vi "Custom Processing.vi"(0 "tagged llp packets cluster in":T1, 1 "reset":bool, 5 "end of data":bool[](array[boolean])=[FALSE, TRUE, TRUE, TRUE, TRUE, TRUE, TRUE, TRUE], 9 "input valid":bool[](array[boolean])=[FALSE, FALSE, FALSE, FALSE, FALSE, FALSE, FALSE, FALSE], 12 "ready for output":bool[](array[boolean])=[TRUE, TRUE, TRUE, TRUE, TRUE, TRUE, TRUE, TRUE]) -> (4 "tagged llp packets cluster out":T1, 6 "end of data out":bool[](array[boolean]), 10 "output valid":bool[](array[boolean]), 14 "ready for input":bool[](array[boolean]))   [LabVIEW 2020, in "GettingStarted_Gen_148X_FPGA.lvlib"]
uses:
  GettingStarted_Gen_148X_FPGA.lvlib
  Common/Types/Tagged LLP Packets Cluster.ctl
  <instrlib>/FlexRIO/CSI-2/v2/FPGA/Types/Tagged LLP Packet.ctl
  <instrlib>/FlexRIO/CSI-2/v2/FPGA/Types/FPGA LLP Packet Tag.ctl
  <instrlib>/FlexRIO/CSI-2/v2/FPGA/Types/FPGA LLP Packet Timestamp.ctl
  <instrlib>/FlexRIO/CSI-2/v2/FPGA/Types/Timestamp ID.ctl
  <instrlib>/FlexRIO/CSI-2/v2/FPGA/Types/FPGA LLP Packet Size.ctl
  <instrlib>/FlexRIO/CSI-2/v2/FPGA/Types/LLP Packet.ctl
  <instrlib>/FlexRIO/CSI-2/v2/FPGA/Types/LLP Packet Header.ctl
  <instrlib>/FlexRIO/CSI-2/v2/FPGA/Types/LLP Packet Payload.ctl
  <instrlib>/FlexRIO/CSI-2/v2/FPGA/Types/LLP Packet Footer.ctl
  <instrlib>/_niInstr/Basic Elements/v1/FPGA/niInstr Basic Elements v1 FPGA.lvlib
  <instrlib>/FlexRIO/CSI-2/v2/FPGA/NI CSI-2 API FPGA v2.lvlib
  Common/GettingStarted_Common_148X_FPGA.lvlib
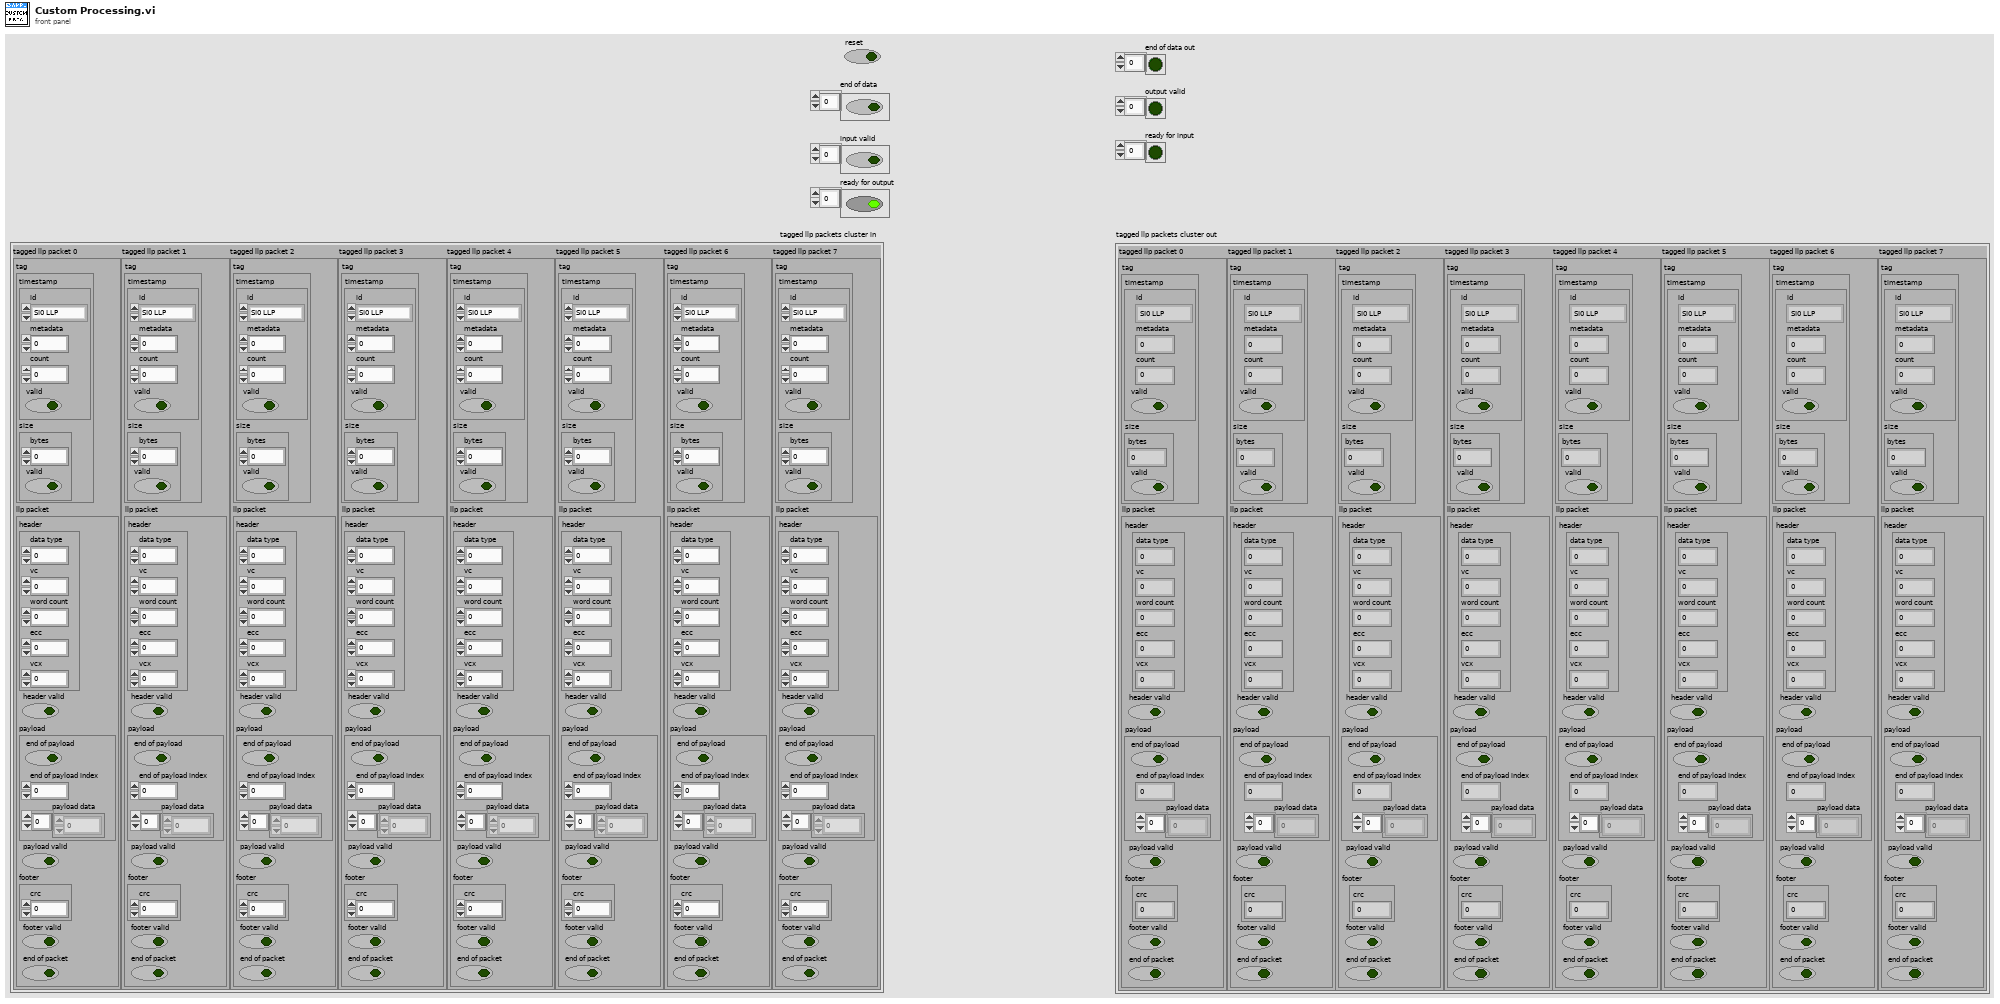
[diagram p1: front panel]
types:
  T1 = typedef "GettingStarted_Common_148X_FPGA.lvlib/Tagged LLP Packets Cluster.ctl" = cluster{"tagged llp packet 0":T2, "tagged llp packet 1":T2, "tagged llp packet 2":T2, "tagged llp packet 3":T2, "tagged llp packet 4":T2, "tagged llp packet 5":T2, "tagged llp packet 6":T2, "tagged llp packet 7":T2}
  T2 = typedef "NI CSI-2 API FPGA v2.lvlib/Tagged LLP Packet.ctl" = cluster{"tag":T3, "llp packet":T7}
  T3 = typedef "NI CSI-2 API FPGA v2.lvlib/FPGA LLP Packet Tag.ctl" = cluster{"timestamp":T4, "size":T6}
  T4 = typedef "NI CSI-2 API FPGA v2.lvlib/FPGA LLP Packet Timestamp.ctl" = cluster{"valid":bool, "count":fxp<+,50,50>, "id":T5, "metadata":u8}
  T5 = typedef "NI CSI-2 API FPGA v2.lvlib/Timestamp ID.ctl" = enum8{"SI0 LLP", "SI1 LLP", "SI2 LLP", "SI3 LLP", "SI4 LLP", "SI5 LLP", "SI6 LLP", "SI7 LLP", "SO0 LLP", "SO1 LLP", "SO2 LLP", "SO3 LLP", "SO4 LLP", "SO5 LLP", "SO6 LLP", "SO7 LLP", "Ser0 GPIO Bank", "Ser1 GPIO Bank", "Ser2 GPIO Bank", "Ser3 GPIO Bank", "Ser4 GPIO Bank", "Ser5 GPIO Bank", "Ser6 GPIO Bank", "Ser7 GPIO Bank", "Des0 GPIO Bank", "Des1 GPIO Bank", "Des2 GPIO Bank", "Des3 GPIO Bank", "Des4 GPIO Bank", "Des5 GPIO Bank", "Des6 GPIO Bank", "Des7 GPIO Bank", "User0", "User1", "User2", "User3", "User4", "User5", "User6", "User7", "User8", "User9", "User10", "User11", "User12", "User13", "User14", "User15", "User16", "User17", "User18", "User19", "User20", "User21", "User22", "User23", "User24", "User25", "User26", "User27", "User28", "User29", "User30", "User31"}
  T6 = typedef "NI CSI-2 API FPGA v2.lvlib/FPGA LLP Packet Size.ctl" = cluster{"bytes":fxp<+,17,17>, "valid":bool}
  T7 = typedef "NI CSI-2 API FPGA v2.lvlib/LLP Packet.ctl" = cluster{"header":T8, "header valid":bool, "payload":T9, "payload valid":bool, "footer":T10, "footer valid":bool, "end of packet":bool}
  T8 = typedef "NI CSI-2 API FPGA v2.lvlib/LLP Packet Header.ctl" = cluster{"word count":u16, "ecc":fxp<+,6,6>, "vcx":fxp<+,2,2>, "data type":fxp<+,6,6>, "vc":fxp<+,2,2>}
  T9 = typedef "NI CSI-2 API FPGA v2.lvlib/LLP Packet Payload.ctl" = cluster{"end of payload":bool, "end of payload index":fxp<+,3,3>, "payload data":u8[]}
  T10 = typedef "NI CSI-2 API FPGA v2.lvlib/LLP Packet Footer.ctl" = cluster{"crc":u16}
  T11 = cluster{"tagged llp packet":T2, "end of data":bool, "input valid":bool, "ready for output":bool}
  T12 = cluster{"end of data out":bool, "output valid":bool, "ready for input":bool}
  T13 = cluster{"end of data out":bool, "output valid":bool, "ready for input":bool}[]
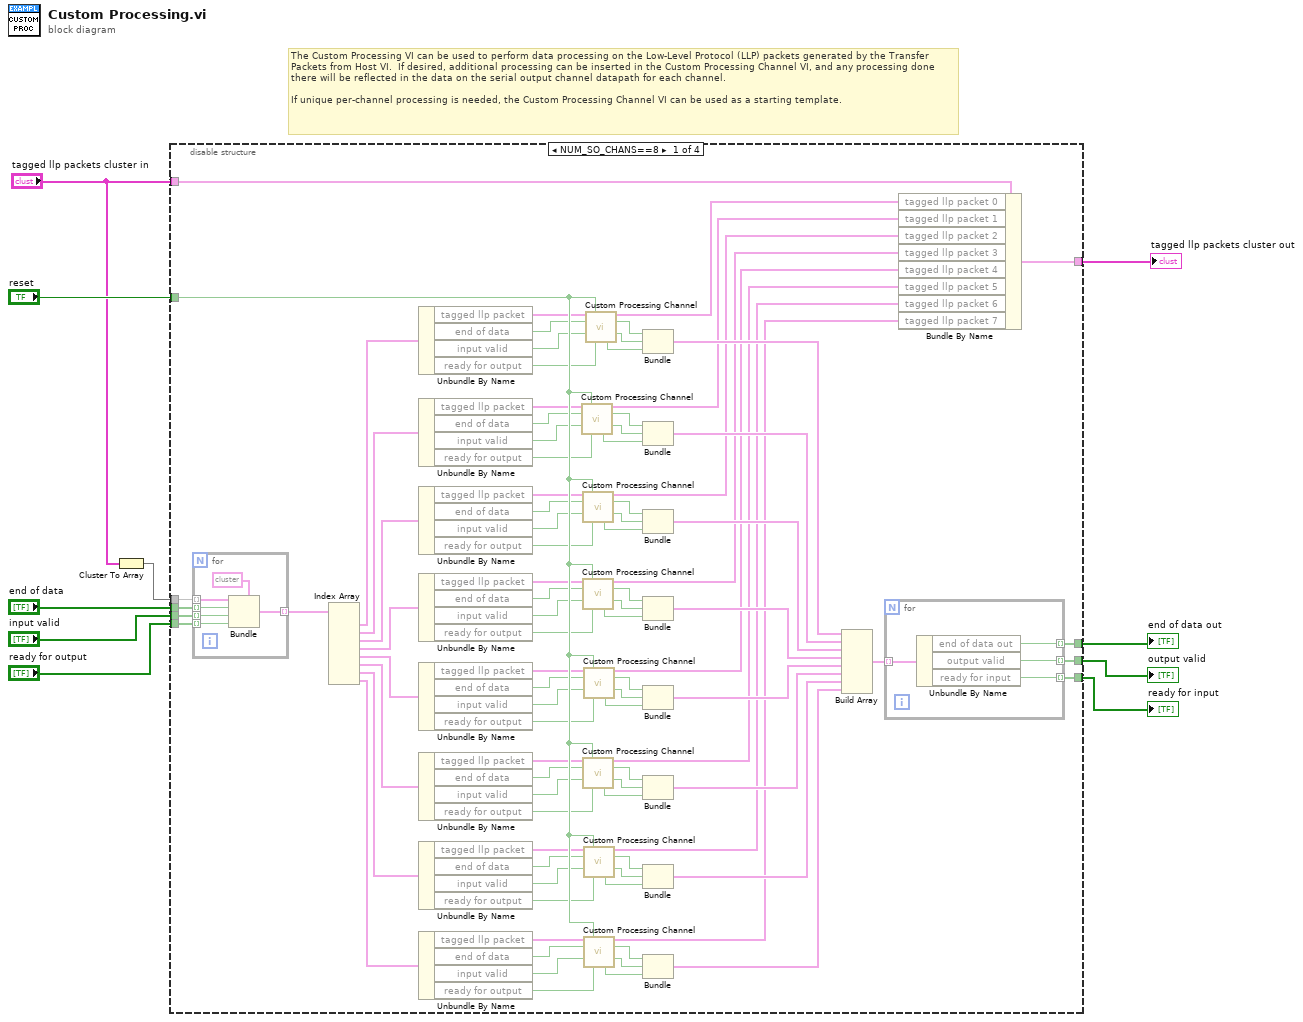
[diagram p0: block diagram]
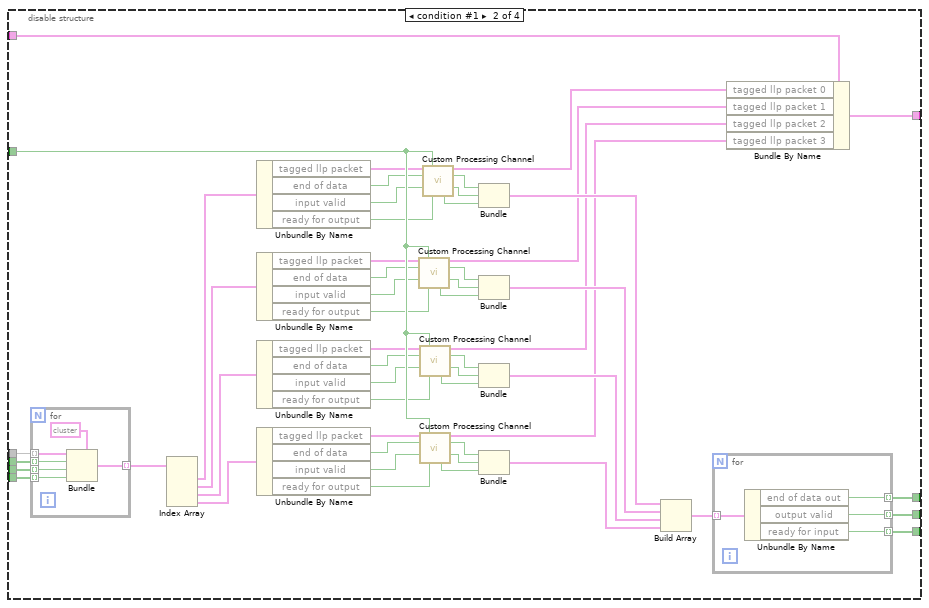
[diagram p2: hidden frame]
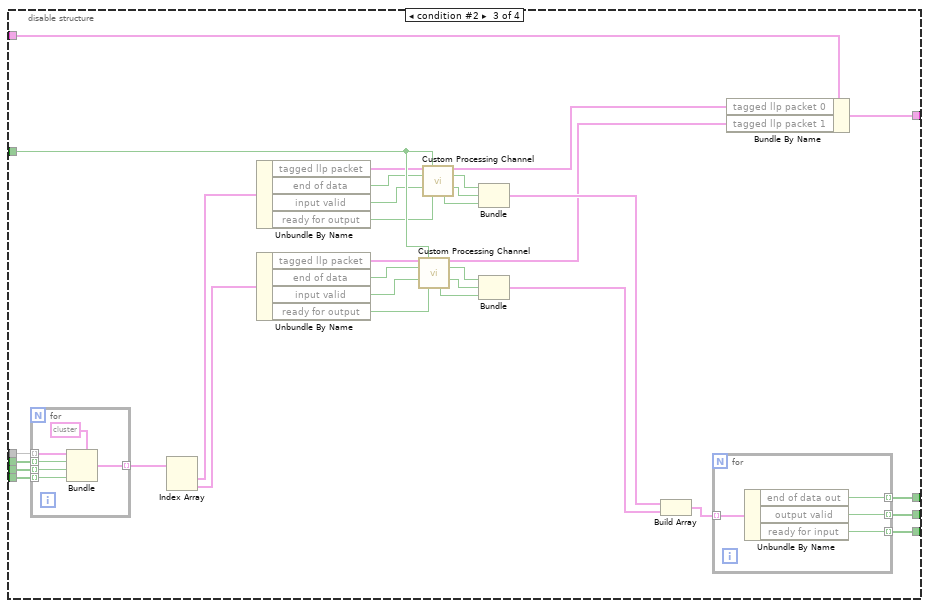
[diagram p3: hidden frame]
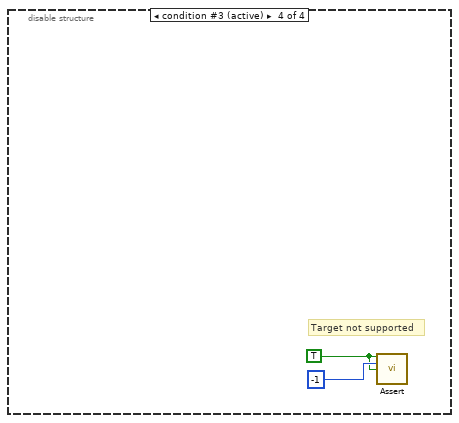
[diagram p4: hidden frame]
diagram:
  # "The Custom Processing VI can be used to perform data processing on the Low-Level Protocol (LLP) packets generated by the Transfer Packets from Host VI.  If desired, additional processing can be inserted in the Custom Processing Channel VI, and any processing done there will be reflected in the data on the serial output channel datapath for each channel.\n\nIf unique per-channel processing is needed, the Custom Processing Channel VI can be used as a starting template."
  n1 = Cluster To Array(cluster="tagged llp packets cluster in") -> (array=w3:T2[])
  n2 = disable-structure shown="NUM_SO_CHANS==8" {
    disable-tunnel: "reset" -> [w91 w158 w202 _]
    disable-tunnel: w3 -> [w102 w114 w176 _]
    disable-tunnel: "end of data" -> [w101 w164 w206 _]
    disable-tunnel: "input valid" -> [w73 w148 w196 _]
    disable-tunnel: "ready for output" -> [w56 w139 w191 _]
    disable-tunnel: [w47 w134 w188 _] -> w4
    disable-tunnel: [w46 w133 w187 _] -> w5
    disable-tunnel: [w21 w120 w180 _] -> w6
    disable-tunnel: [w12 w119 w179 _] -> w2
    disable-tunnel: "tagged llp packets cluster in" -> [w11 w113 w175 _]
    frame condition #0 {
      n3 = for {
        tunnel: w102 -> [w107] mode=indexing
        tunnel: w101 -> [w106] mode=indexing
        tunnel: [w108] -> w100 mode=indexing
        tunnel: w73 -> [w105] mode=indexing
        tunnel: w56 -> [w104] mode=indexing
        n4 = Bundle(cluster=T11 {"tagged llp packet"={"tag"={"timestamp"={"valid"=FALSE, "count"=0.0, "id"=enum."SI0 LLP", "metadata"=0}, "size"={"bytes"=0.0, "valid"=FALSE}}, "llp packet"={"header"={"word count"=0, "ecc"=0.0, "vcx"=0.0, "data type"=0.0, "vc"=0.0}, "header valid"=FALSE, "payload"={"end of payload"=FALSE, "end of payload index"=0.0, "payload data"=[]}, "payload valid"=FALSE, "footer"={"crc"=0}, "footer valid"=FALSE, "end of packet"=FALSE}}, "end of data"=FALSE, "input valid"=FALSE, "ready for output"=FALSE} ("output cluster"), "tagged llp packet"=w107, "end of data"=w106, "input valid"=w105, "ready for output"=w104) -> (w108:T11)
      }
      n5 = Index Array(array=w100) -> (element #1=w99:T11, element #2=w96:T11, element #3=w95:T11, element #4=w93:T11, element #5=w92:T11, element #6=w94:T11, element #7=w97:T11, element #8=w98:T11)  [unwired: 8 in]
      n6 = Unbundle By Name(w99) -> ("tagged llp packet"=w90:T2, "end of data"=w71:bool, "input valid"=w72:bool, "ready for output"=w55:bool)
      n7 = Unbundle By Name(w96) -> ("tagged llp packet"=w89:T2, "end of data"=w70:bool, "input valid"=w69:bool, "ready for output"=w54:bool)
      n8 = Unbundle By Name(w95) -> ("tagged llp packet"=w83:T2, "end of data"=w68:bool, "input valid"=w67:bool, "ready for output"=w53:bool)
      n9 = Unbundle By Name(w93) -> ("tagged llp packet"=w84:T2, "end of data"=w66:bool, "input valid"=w65:bool, "ready for output"=w52:bool)
      n10 = Unbundle By Name(w92) -> ("tagged llp packet"=w85:T2, "end of data"=w64:bool, "input valid"=w63:bool, "ready for output"=w51:bool)
      n11 = Unbundle By Name(w94) -> ("tagged llp packet"=w86:T2, "end of data"=w62:bool, "input valid"=w61:bool, "ready for output"=w50:bool)
      n12 = Unbundle By Name(w97) -> ("tagged llp packet"=w87:T2, "end of data"=w60:bool, "input valid"=w59:bool, "ready for output"=w49:bool)
      n13 = Unbundle By Name(w98) -> ("tagged llp packet"=w88:T2, "end of data"=w58:bool, "input valid"=w57:bool, "ready for output"=w48:bool)
      n14 = call "Custom Processing Channel.vi"("tagged llp packet in"=w89, "reset"=w91, "end of data in"=w70, "input valid"=w69, "ready for output"=w54) -> ("tagged llp packet out"=w14:T2, "end of data out"=w25:bool, "output valid"=w26:bool, "ready for input"=w44:bool)  [unwired: 7 in]
      n15 = call "Custom Processing Channel.vi"("tagged llp packet in"=w83, "reset"=w91, "end of data in"=w68, "input valid"=w67, "ready for output"=w53) -> ("tagged llp packet out"=w15:T2, "end of data out"=w28:bool, "output valid"=w27:bool, "ready for input"=w45:bool)  [unwired: 7 in]
      n16 = call "Custom Processing Channel.vi"("tagged llp packet in"=w84, "reset"=w91, "end of data in"=w66, "input valid"=w65, "ready for output"=w52) -> ("tagged llp packet out"=w16:T2, "end of data out"=w29:bool, "output valid"=w30:bool, "ready for input"=w42:bool)  [unwired: 7 in]
      n17 = call "Custom Processing Channel.vi"("tagged llp packet in"=w86, "reset"=w91, "end of data in"=w62, "input valid"=w61, "ready for output"=w50) -> ("tagged llp packet out"=w18:T2, "end of data out"=w33:bool, "output valid"=w34:bool, "ready for input"=w40:bool)  [unwired: 7 in]
      n18 = call "Custom Processing Channel.vi"("tagged llp packet in"=w85, "reset"=w91, "end of data in"=w64, "input valid"=w63, "ready for output"=w51) -> ("tagged llp packet out"=w17:T2, "end of data out"=w32:bool, "output valid"=w31:bool, "ready for input"=w41:bool)  [unwired: 7 in]
      n19 = call "Custom Processing Channel.vi"("tagged llp packet in"=w87, "reset"=w91, "end of data in"=w60, "input valid"=w59, "ready for output"=w49) -> ("tagged llp packet out"=w19:T2, "end of data out"=w22:bool, "output valid"=w37:bool, "ready for input"=w39:bool)  [unwired: 7 in]
      n20 = call "Custom Processing Channel.vi"("tagged llp packet in"=w88, "reset"=w91, "end of data in"=w58, "input valid"=w57, "ready for output"=w48) -> ("tagged llp packet out"=w20:T2, "end of data out"=w35:bool, "output valid"=w36:bool, "ready for input"=w38:bool)  [unwired: 7 in]
      n21 = call "Custom Processing Channel.vi"("tagged llp packet in"=w90, "reset"=w91, "end of data in"=w71, "input valid"=w72, "ready for output"=w55) -> ("tagged llp packet out"=w13:T2, "end of data out"=w23:bool, "output valid"=w24:bool, "ready for input"=w43:bool)  [unwired: 7 in]
      n22 = Bundle("end of data out"=w23, "output valid"=w24, "ready for input"=w43) -> (w80:T12)  [unwired: 1 in]
      n23 = Bundle("end of data out"=w25, "output valid"=w26, "ready for input"=w44) -> (w77:T12)  [unwired: 1 in]
      n24 = Bundle("end of data out"=w28, "output valid"=w27, "ready for input"=w45) -> (w76:T12)  [unwired: 1 in]
      n25 = Bundle("end of data out"=w29, "output valid"=w30, "ready for input"=w42) -> (w82:T12)  [unwired: 1 in]
      n26 = Bundle("end of data out"=w32, "output valid"=w31, "ready for input"=w41) -> (w81:T12)  [unwired: 1 in]
      n27 = Bundle("end of data out"=w33, "output valid"=w34, "ready for input"=w40) -> (w75:T12)  [unwired: 1 in]
      n28 = Bundle("end of data out"=w22, "output valid"=w37, "ready for input"=w39) -> (w78:T12)  [unwired: 1 in]
      n29 = Bundle("end of data out"=w35, "output valid"=w36, "ready for input"=w38) -> (w79:T12)  [unwired: 1 in]
      n30 = Build Array(w80, w77, w76, w82, w81, w75, w78, w79) -> (w74:T13)
      n31 = for {
        tunnel: w74 -> [w112] mode=indexing
        tunnel: [w111] -> w47 mode=indexing
        tunnel: [w110] -> w46 mode=indexing
        tunnel: [w109] -> w21 mode=indexing
        n32 = Unbundle By Name(w112) -> ("end of data out"=w111:bool, "output valid"=w110:bool, "ready for input"=w109:bool)
      }
      n33 = Bundle By Name(cluster=w11, "tagged llp packet 0"=w13, "tagged llp packet 1"=w14, "tagged llp packet 2"=w15, "tagged llp packet 3"=w16, "tagged llp packet 4"=w17, "tagged llp packet 5"=w18, "tagged llp packet 6"=w19, "tagged llp packet 7"=w20) -> (w12:T1)
    }
    frame condition #1 {
      n34 = for {
        tunnel: w114 -> [w169] mode=indexing
        tunnel: w164 -> [w168] mode=indexing
        tunnel: [w170] -> w163 mode=indexing
        tunnel: w148 -> [w167] mode=indexing
        tunnel: w139 -> [w166] mode=indexing
        n35 = Bundle(cluster=T11 {"tagged llp packet"={"tag"={"timestamp"={"valid"=FALSE, "count"=0.0, "id"=enum."SI0 LLP", "metadata"=0}, "size"={"bytes"=0.0, "valid"=FALSE}}, "llp packet"={"header"={"word count"=0, "ecc"=0.0, "vcx"=0.0, "data type"=0.0, "vc"=0.0}, "header valid"=FALSE, "payload"={"end of payload"=FALSE, "end of payload index"=0.0, "payload data"=[]}, "payload valid"=FALSE, "footer"={"crc"=0}, "footer valid"=FALSE, "end of packet"=FALSE}}, "end of data"=FALSE, "input valid"=FALSE, "ready for output"=FALSE} ("output cluster"), "tagged llp packet"=w169, "end of data"=w168, "input valid"=w167, "ready for output"=w166) -> (w170:T11)
      }
      n36 = Index Array(array=w163) -> (element #1=w162:T11, element #2=w161:T11, element #3=w160:T11, element #4=w159:T11)  [unwired: 4 in]
      n37 = Unbundle By Name(w162) -> ("tagged llp packet"=w157:T2, "end of data"=w146:bool, "input valid"=w147:bool, "ready for output"=w138:bool)
      n38 = Unbundle By Name(w161) -> ("tagged llp packet"=w156:T2, "end of data"=w145:bool, "input valid"=w144:bool, "ready for output"=w137:bool)
      n39 = Unbundle By Name(w160) -> ("tagged llp packet"=w154:T2, "end of data"=w143:bool, "input valid"=w142:bool, "ready for output"=w136:bool)
      n40 = Unbundle By Name(w159) -> ("tagged llp packet"=w155:T2, "end of data"=w141:bool, "input valid"=w140:bool, "ready for output"=w135:bool)
      n41 = call "Custom Processing Channel.vi"("tagged llp packet in"=w156, "reset"=w158, "end of data in"=w145, "input valid"=w144, "ready for output"=w137) -> ("tagged llp packet out"=w116:T2, "end of data out"=w123:bool, "output valid"=w124:bool, "ready for input"=w131:bool)  [unwired: 7 in]
      n42 = call "Custom Processing Channel.vi"("tagged llp packet in"=w154, "reset"=w158, "end of data in"=w143, "input valid"=w142, "ready for output"=w136) -> ("tagged llp packet out"=w117:T2, "end of data out"=w126:bool, "output valid"=w125:bool, "ready for input"=w132:bool)  [unwired: 7 in]
      n43 = call "Custom Processing Channel.vi"("tagged llp packet in"=w155, "reset"=w158, "end of data in"=w141, "input valid"=w140, "ready for output"=w135) -> ("tagged llp packet out"=w118:T2, "end of data out"=w127:bool, "output valid"=w128:bool, "ready for input"=w129:bool)  [unwired: 7 in]
      n44 = call "Custom Processing Channel.vi"("tagged llp packet in"=w157, "reset"=w158, "end of data in"=w146, "input valid"=w147, "ready for output"=w138) -> ("tagged llp packet out"=w115:T2, "end of data out"=w121:bool, "output valid"=w122:bool, "ready for input"=w130:bool)  [unwired: 7 in]
      n45 = Bundle("end of data out"=w121, "output valid"=w122, "ready for input"=w130) -> (w152:T12)  [unwired: 1 in]
      n46 = Bundle("end of data out"=w123, "output valid"=w124, "ready for input"=w131) -> (w151:T12)  [unwired: 1 in]
      n47 = Bundle("end of data out"=w126, "output valid"=w125, "ready for input"=w132) -> (w150:T12)  [unwired: 1 in]
      n48 = Bundle("end of data out"=w127, "output valid"=w128, "ready for input"=w129) -> (w153:T12)  [unwired: 1 in]
      n49 = Build Array(w152, w151, w150, w153) -> (w149:T13)
      n50 = for {
        tunnel: w149 -> [w174] mode=indexing
        tunnel: [w173] -> w134 mode=indexing
        tunnel: [w172] -> w133 mode=indexing
        tunnel: [w171] -> w120 mode=indexing
        n51 = Unbundle By Name(w174) -> ("end of data out"=w173:bool, "output valid"=w172:bool, "ready for input"=w171:bool)
      }
      n52 = Bundle By Name(cluster=w113, "tagged llp packet 0"=w115, "tagged llp packet 1"=w116, "tagged llp packet 2"=w117, "tagged llp packet 3"=w118) -> (w119:T1)
    }
    frame condition #2 {
      n53 = for {
        tunnel: w176 -> [w211] mode=indexing
        tunnel: w206 -> [w210] mode=indexing
        tunnel: [w212] -> w205 mode=indexing
        tunnel: w196 -> [w209] mode=indexing
        tunnel: w191 -> [w208] mode=indexing
        n54 = Bundle(cluster=T11 {"tagged llp packet"={"tag"={"timestamp"={"valid"=FALSE, "count"=0.0, "id"=enum."SI0 LLP", "metadata"=0}, "size"={"bytes"=0.0, "valid"=FALSE}}, "llp packet"={"header"={"word count"=0, "ecc"=0.0, "vcx"=0.0, "data type"=0.0, "vc"=0.0}, "header valid"=FALSE, "payload"={"end of payload"=FALSE, "end of payload index"=0.0, "payload data"=[]}, "payload valid"=FALSE, "footer"={"crc"=0}, "footer valid"=FALSE, "end of packet"=FALSE}}, "end of data"=FALSE, "input valid"=FALSE, "ready for output"=FALSE} ("output cluster"), "tagged llp packet"=w211, "end of data"=w210, "input valid"=w209, "ready for output"=w208) -> (w212:T11)
      }
      n55 = Index Array(array=w205) -> (element #1=w204:T11, element #2=w203:T11)  [unwired: 2 in]
      n56 = Unbundle By Name(w204) -> ("tagged llp packet"=w201:T2, "end of data"=w194:bool, "input valid"=w195:bool, "ready for output"=w190:bool)
      n57 = Unbundle By Name(w203) -> ("tagged llp packet"=w200:T2, "end of data"=w193:bool, "input valid"=w192:bool, "ready for output"=w189:bool)
      n58 = call "Custom Processing Channel.vi"("tagged llp packet in"=w200, "reset"=w202, "end of data in"=w193, "input valid"=w192, "ready for output"=w189) -> ("tagged llp packet out"=w178:T2, "end of data out"=w183:bool, "output valid"=w184:bool, "ready for input"=w186:bool)  [unwired: 7 in]
      n59 = call "Custom Processing Channel.vi"("tagged llp packet in"=w201, "reset"=w202, "end of data in"=w194, "input valid"=w195, "ready for output"=w190) -> ("tagged llp packet out"=w177:T2, "end of data out"=w181:bool, "output valid"=w182:bool, "ready for input"=w185:bool)  [unwired: 7 in]
      n60 = Bundle("end of data out"=w181, "output valid"=w182, "ready for input"=w185) -> (w199:T12)  [unwired: 1 in]
      n61 = Bundle("end of data out"=w183, "output valid"=w184, "ready for input"=w186) -> (w198:T12)  [unwired: 1 in]
      n62 = Build Array(w199, w198) -> (w197:T13)
      n63 = for {
        tunnel: w197 -> [w216] mode=indexing
        tunnel: [w215] -> w188 mode=indexing
        tunnel: [w214] -> w187 mode=indexing
        tunnel: [w213] -> w180 mode=indexing
        n64 = Unbundle By Name(w216) -> ("end of data out"=w215:bool, "output valid"=w214:bool, "ready for input"=w213:bool)
      }
      n65 = Bundle By Name(cluster=w175, "tagged llp packet 0"=w177, "tagged llp packet 1"=w178) -> (w179:T1)
    }
    frame condition #3 (active) {
      w217 = TRUE ("assert")
      # "Target not supported"
      n66 = call <instrlib>:"Assert.vi"("assert"=w217, "error code"=-1, "enable show error"=w217) -> ()  [unwired: 13 in]
    }
  }
  "output valid" <- w5
  "ready for input" <- w6
  "end of data out" <- w4
  "tagged llp packets cluster out" <- w2
